vi "Unflatten-JoyBatteryEventData.vi"(8 "error in (no error)":errorcluster, 11 "Event Binary Data":string) -> (0 "error out":errorcluster, 3 "Event Data":T1 {"State" items=["SDL_POWERSTATE_ERROR"=-1, "SDL_POWERSTATE_UNKNOWN"=0, "SDL_POWERSTATE_ON_BATTERY"=1, "SDL_POWERSTATE_NO_BATTERY"=2, "SDL_POWERSTATE_CHARGING"=3, "SDL_POWERSTATE_CHARGED       "=4]})   [LabVIEW 2026, in "SDL3.lvlib" / "Events.lvlib"]
uses:
  JoyBatteryEventData--cluster.ctl
  Joystick/JoystickID--integer.ctl
  Power/PowerState--ring.ctl
  Events.lvlib
  Joystick/Joystick.lvlib
  Power/Power.lvlib
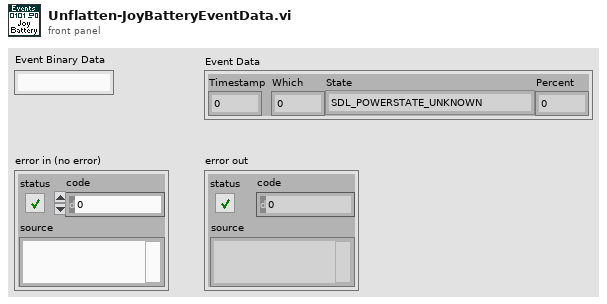
[diagram p1: front panel]
types:
  T1 = typedef "SDL3.lvlib/Events.lvlib/JoyBatteryEventData--cluster.ctl" = cluster{"Timestamp":u64, "Which":T2, "State":T3, "Percent":i32}
  T2 = typedef "SDL3.lvlib/Joystick.lvlib/JoystickID--integer.ctl" = u32
  T3 = typedef "SDL3.lvlib/Power.lvlib/PowerState--ring.ctl" = i32
  T4 = enum16{"big-endian, network order", "native, host order", "little-endian"}
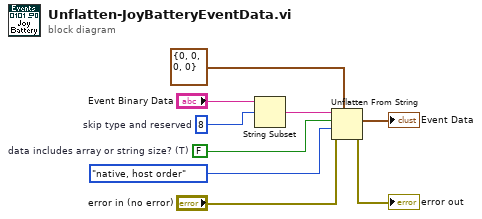
[diagram p0: block diagram]
diagram:
  w3 = 8  # skip type and reserved
  w6 = FALSE  # data includes array or string size? (T)
  n1 = String Subset(string="Event Binary Data", offset (0)=w3) -> (substring=w4:string)  [unwired: 1 in]
  n2 = Unflatten From String(type=T1 {"Timestamp"=0, "Which"=0, "State"=0, "Percent"=0} ("JoyBatteryEvent"), binary string=w4, data includes array or string size? (T)=w6, byte order (0:big-endian, network order)=T4."native, host order", error in (no error)="error in (no error)") -> (value=→"Event Data":T1, error out=→"error out":errorcluster)  [unwired: 1 out]
